vi "Welcome.vi"() -> ()   [LabVIEW 2023]
uses:
  Global/Global 1.vi
  Global/Login Details.vi
  Control/WELCOM SCREEN ENUM.ctl
panel:
  in  "Check 2":bool
  in  "auto":bool
  in  "Test Print":bool
  in  "andon":bool
  in  "MANUAL":bool
  out "error out 2":errorcluster
  in  "error in (no error) 3":errorcluster
  in  "Remove":bool
  in  "Check":bool
  in  "Home":bool
  out "user name":string
  out "STOP":bool
  in  "Tab Control":enum32{"Page 1", "user mangement"}(tab)
  out "Screen Index":i32
  out "error out":errorcluster
  in  "error in (no error)":errorcluster
  in  "LOGIN":bool
  in  "RECIPE":bool
  in  "EXIT":bool
  in  "REPORT":bool
  in  "Hardware Setting":bool
  in  "Shift Setting":bool
  in  "AUTO MODE":bool
  in  "USER MANGMENT":bool
  out "datetime":string
  # "PV Clean Mobility Technologies Traceability System"
  # "USER :"
  # "Powered By - NiVision Automation Systems Pvt. Ltd."
  # "Powered By-Infinity Automation Systems Pvt Ltd. Pune"
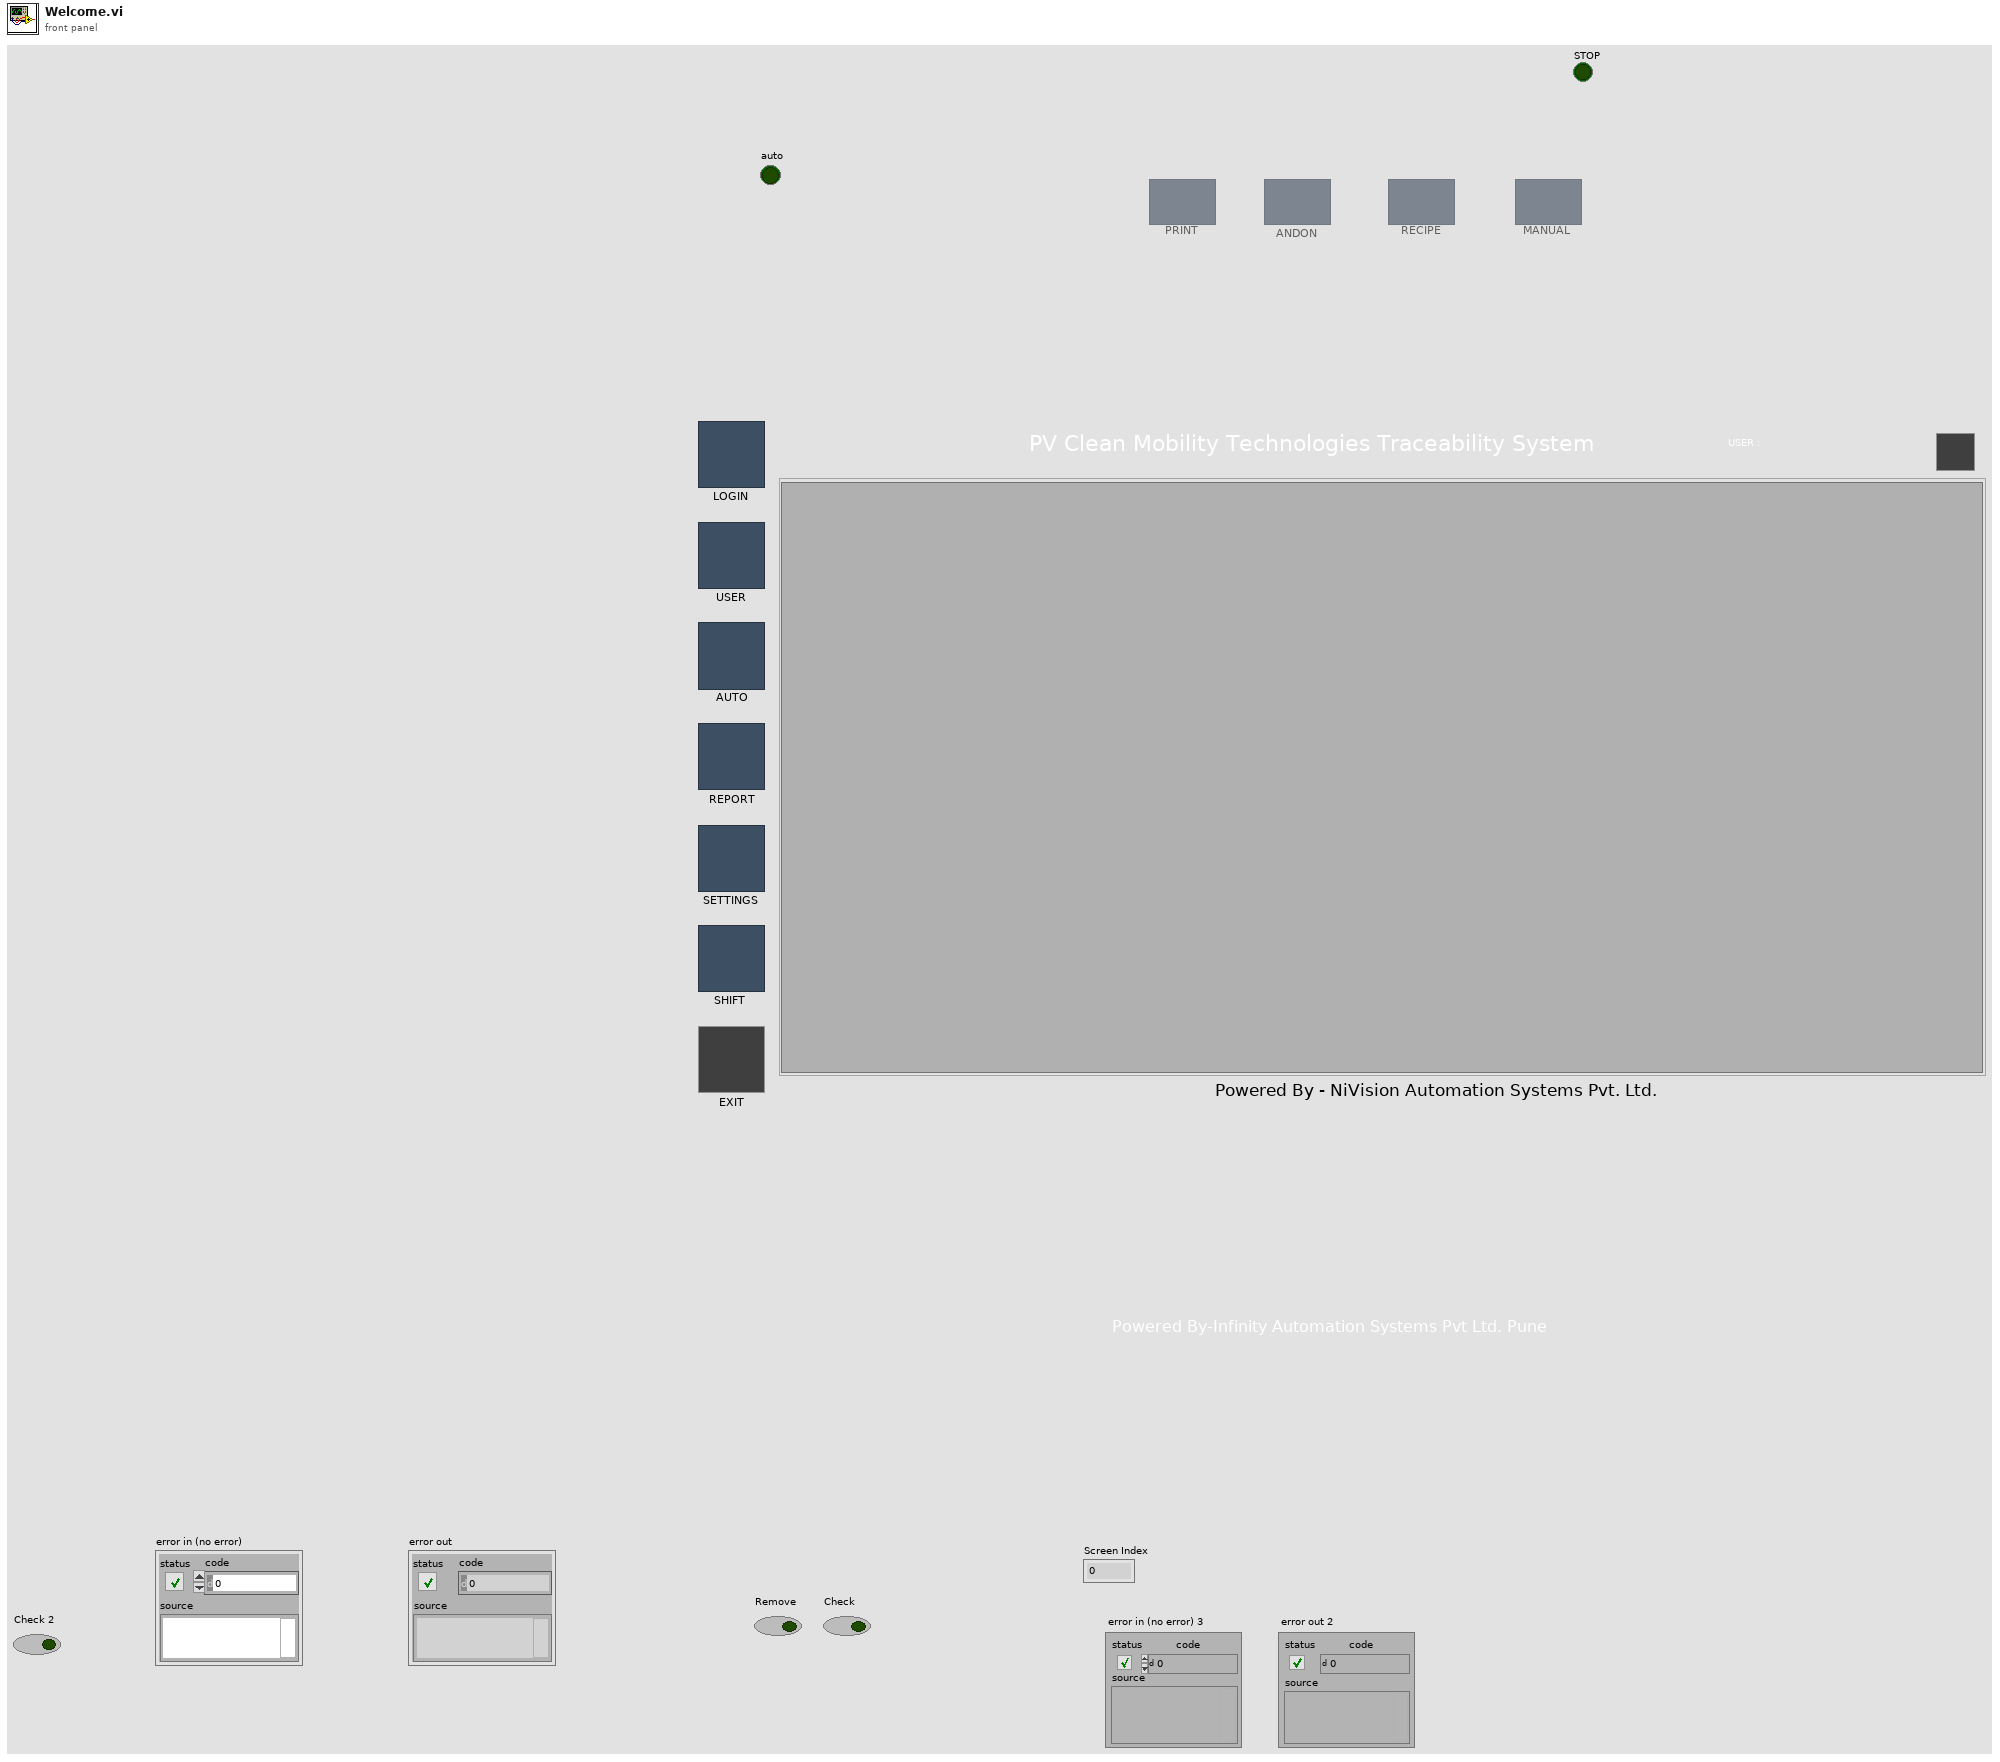
[diagram p1: front panel]
types:
  T1 = typedef "WELCOM SCREEN ENUM.ctl" = enum16{"Initialization", "Wait For Event", "RUN", "LOGIN", "USER MANAGEMENT", "AUTORITY MANAGEMENT", "AUTO MODE", "MANUAL MODE", "BIN MASTER", "CHEMICAL MASTER", "RAW MATERIAL INWARD", "RECIPE INGREDIENT", "REPORT", "SHIFT SETTING", "HARDWARE SETTING", "Check Authority", "TEST PRINT", "EXIT"}
  T2 = cluster{"SCREEN 1":bool, "SCREEN 2":bool, "SCREEN 3":bool, "SCREEN 4":bool, "SCREEN 5":bool, "SCREEN 6":bool, "SCREEN 7":bool, "SCREEN 8":bool, "SCREEN 9":bool, "SCREEN 10":bool, "SCREEN 11":bool, "SCREEN 12":bool, "SCREEN 13":bool, "SCREEN 14":bool, "SCREEN 15":bool, "SCREEN 16":bool, "SCREEN 17":bool, "SCREEN 18":bool, "SCREEN 19":bool, "SCREEN 20":bool}
  T3 = enum8{"Enabled", "Disabled", "Disabled and Grayed Out"}
  T4 = enum32{"Invalid", "Standard", "Closed", "Hidden", "Minimized", "Maximized"}
  T5 = enum32{"Bad", "Idle", "Run top level", "Running"}
  T6 = enum32{"invalid app kind", "Development System", "Run Time System", "Student Edition", "Embedded LabVIEW", "Evaluation", "Custom"}
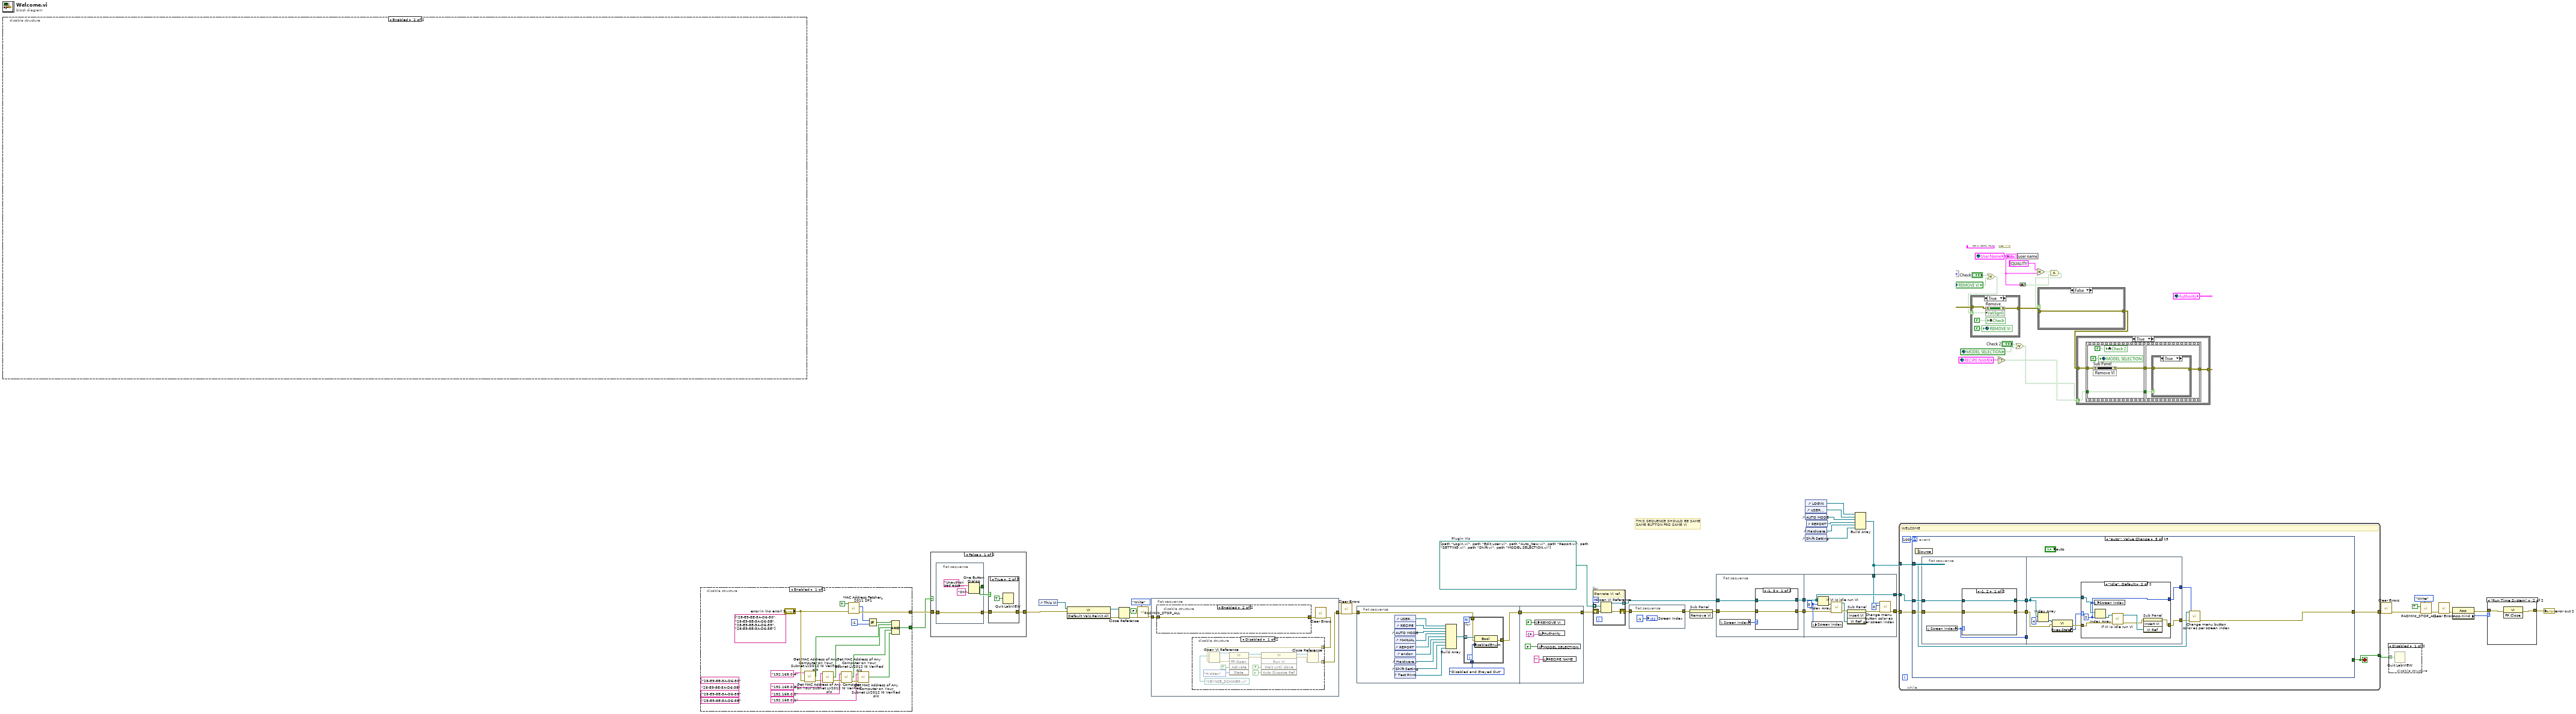
[diagram p0: block diagram]
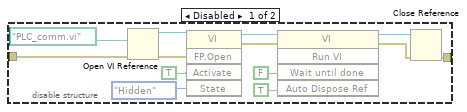
[diagram p2: hidden frame]
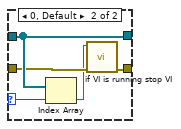
[diagram p4: hidden frame]
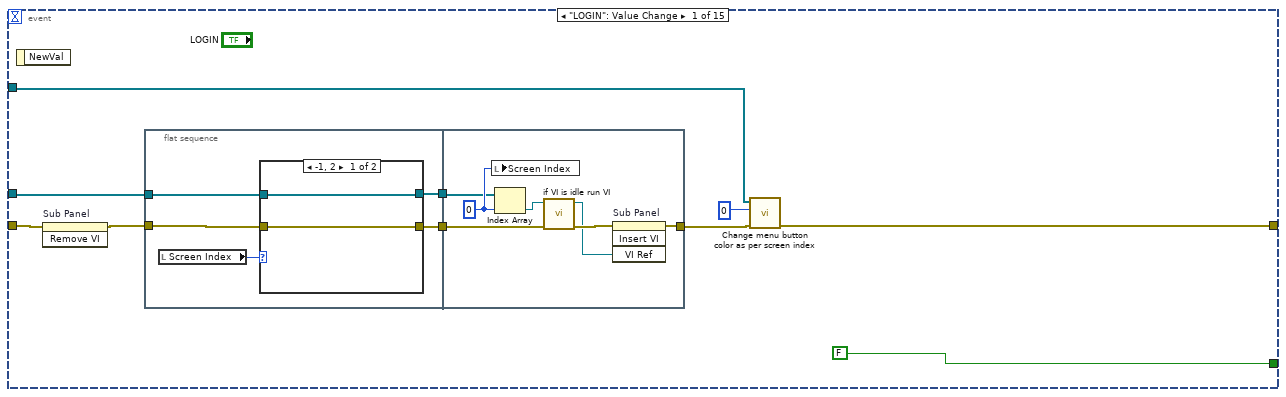
[diagram p7: hidden frame]
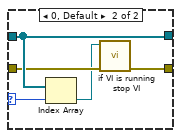
[diagram p8: hidden frame]
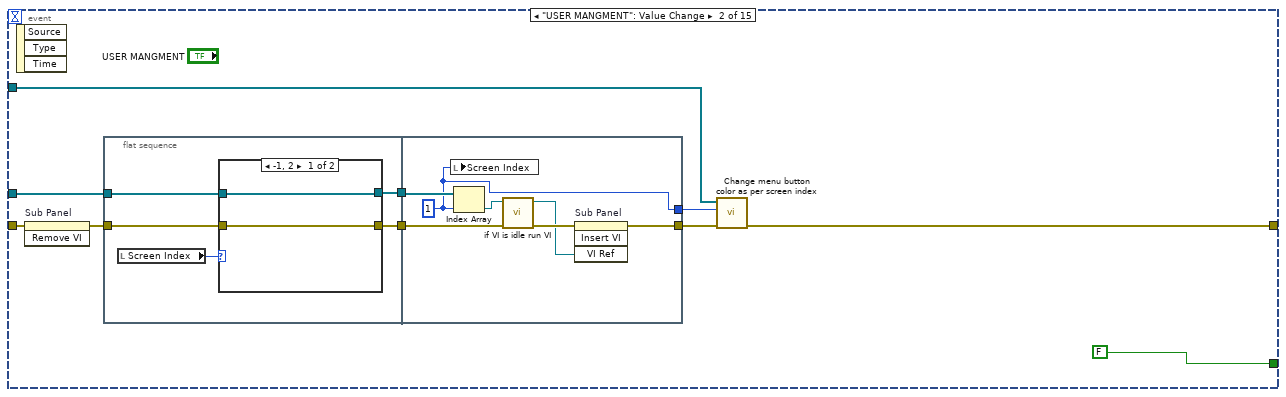
[diagram p9: hidden frame]
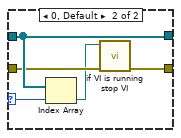
[diagram p10: hidden frame]
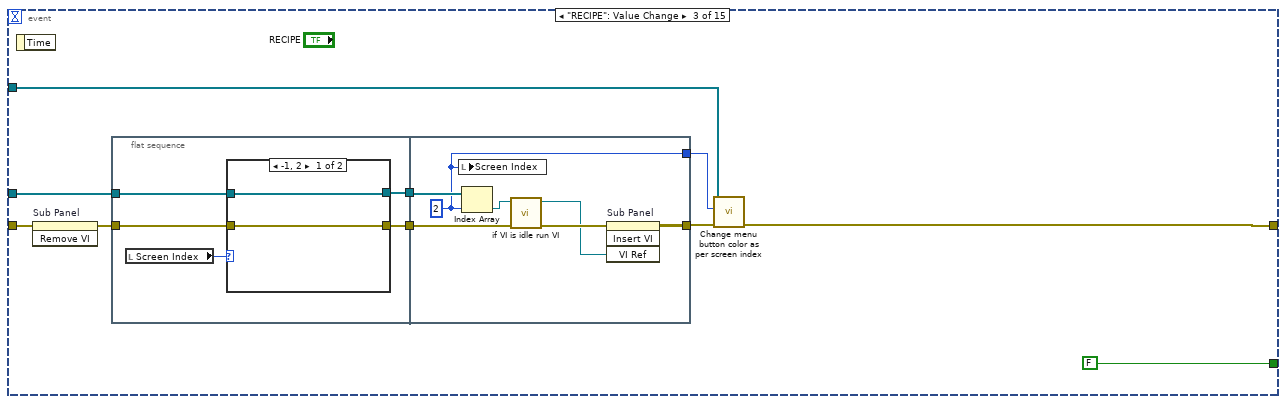
[diagram p11: hidden frame]
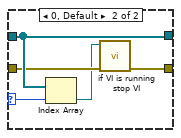
[diagram p12: hidden frame]
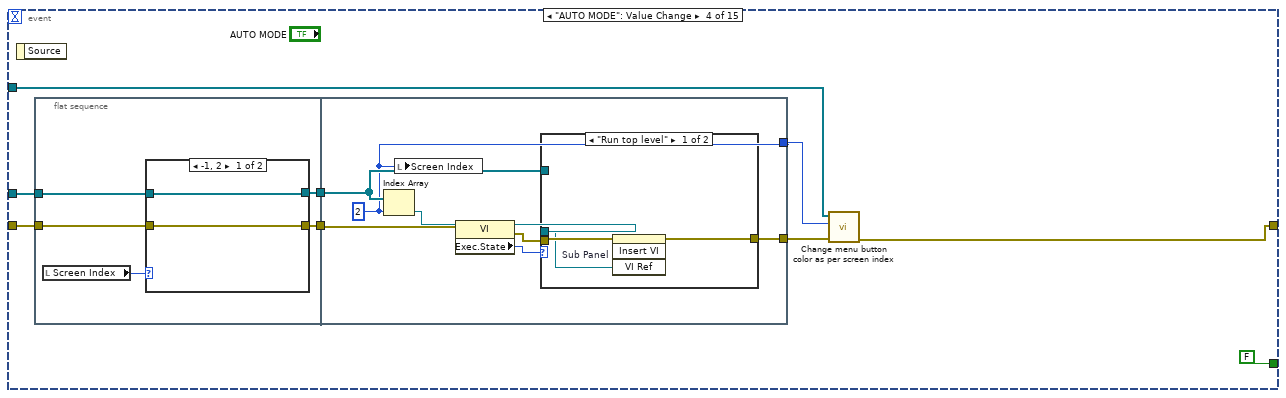
[diagram p13: hidden frame]
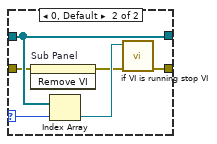
[diagram p14: hidden frame]
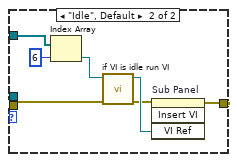
[diagram p15: hidden frame]
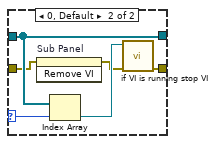
[diagram p16: hidden frame]
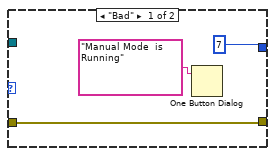
[diagram p17: hidden frame]
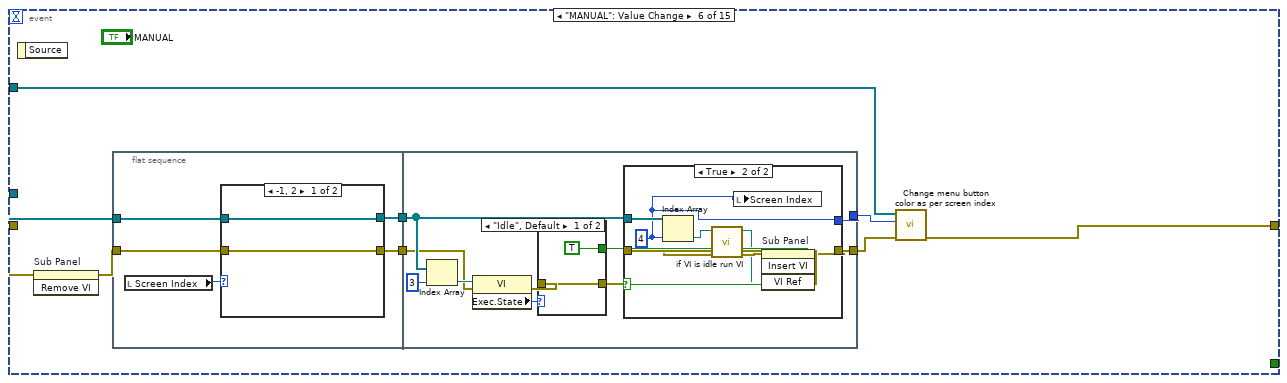
[diagram p18: hidden frame]
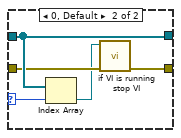
[diagram p19: hidden frame]
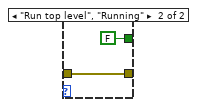
[diagram p20: hidden frame]
diagram:
  w33 = path[] [path "Login.vi", path "Edit user.vi", path "Auto_New.vi", path "Report.vi", path "SETTING.vi", path "Shift.vi", path "MODEL SELECTION.vi"]  # Plugin VIs
  # "THIS SEQUENCE SHOULD BE SAME\nSAME BUTTON FRO SAME VI"
  # "THIS SEQUENCE SHOULD BE SAME\nSAME BUTTON FRO SAME VI"
  n1 = disable-structure shown="Enabled" {
    frame Disabled {
      n2 = flat-sequence {
        tunnel: "error in (no error)" -> [w68]
        tunnel: [w67] -> w43
        frame #0 {
          n3 = invoke class="VI" method="Default Vals.Reinit All"(error in=w68) -> (error out=w67:errorcluster)  [unwired: 2 in, 2 out]
          n4 = global write "Login Details.vi" "Authority"(T2 {"SCREEN 1"=FALSE, "SCREEN 2"=FALSE, "SCREEN 3"=FALSE, "SCREEN 4"=FALSE, "SCREEN 5"=FALSE, "SCREEN 6"=FALSE, "SCREEN 7"=FALSE, "SCREEN 8"=FALSE, "SCREEN 9"=FALSE, "SCREEN 10"=FALSE, "SCREEN 11"=FALSE, "SCREEN 12"=FALSE, "SCREEN 13"=FALSE, "SCREEN 14"=FALSE, "SCREEN 15"=FALSE, "SCREEN 16"=FALSE, "SCREEN 17"=FALSE, "SCREEN 18"=FALSE, "SCREEN 19"=FALSE, "SCREEN 20"=FALSE} ("Authority")) -> ()
        }
      }
      n5 = invoke on="Sub Panel" class="SubPnl" method="Remove VI"(error in=w43) -> (error out=w56:errorcluster)  [unwired: 2 in, 2 out]
      n6 = Open VI Reference(vi path=path "Login.vi", error in (no error)=w56) -> (vi reference=w55:refnum<vi>, error out=w53:errorcluster)  [unwired: 4 in]
      n7 = invoke on="Sub Panel" class="SubPnl" method="Insert VI"(error in=w53, "VI Ref"=w55) -> (error out=w54:errorcluster)  [unwired: 2 in, 3 out]
      n8 = invoke class="VI" method="Run VI"(reference=w55, error in=w54, "Wait until done"=TRUE ("Wait Until Done"), "Auto Dispose Ref"=FALSE ("Auto Dispose Reference")) -> (reference out=w51:refnum<vi>, error out=w52:errorcluster)  [unwired: 1 in, 3 out]
      n9 = Close Reference(reference=w51, error in (no error)=w52) -> (error out=w46:errorcluster)
      n10 = Unbundle By Name(w46) -> ("code"=w50:i32)
      n11 = call <vilib>:"Clear Errors.vi"("error in (no error)"=w46) -> ("error out"=w48:errorcluster)  [unwired: 5 in, 1 out]
      n12 = Not Equal?(x=7, y=w50) -> (x != y?=w49:bool)
      n13 = Select(t=w46, s=w49, f=w48) -> (s? t:f=w47:errorcluster)
      n14 = call <vilib>:"Simple Error Handler.vi"("error in (no error)"=w47) -> ("error out"=w57:errorcluster)  [unwired: 4 in, 4 out]
      n15 = invoke on="Sub Panel" class="SubPnl" method="Remove VI"(error in=w57) -> (error out=w45:errorcluster)  [unwired: 2 in, 2 out]
      n16 = while {
        tunnel: w45 -> [w75]
        shift-right: [w77] -> _
        shift-left: WELCOM_SCREEN_ENUM."Initialization" -> [w71]
        shift-right: [w74] -> _
        shift-left: cluster{"VI Run":string} {"VI Run"=""} -> [w73]
        tunnel: [w76] -> w63
        stop <- w72 stop-if-true
        n17 = case shown="\"AUTORITY MANAGEMENT\"" w71 {
          tunnel: [WELCOM_SCREEN_ENUM."Check Authority" w102 WELCOM_SCREEN_ENUM."Wait For Event" WELCOM_SCREEN_ENUM."Wait For Event" WELCOM_SCREEN_ENUM."RUN" WELCOM_SCREEN_ENUM."RUN" WELCOM_SCREEN_ENUM."RUN" WELCOM_SCREEN_ENUM."RUN" WELCOM_SCREEN_ENUM."RUN" WELCOM_SCREEN_ENUM."RUN" WELCOM_SCREEN_ENUM."RUN" WELCOM_SCREEN_ENUM."RUN" WELCOM_SCREEN_ENUM."RUN" WELCOM_SCREEN_ENUM."RUN" WELCOM_SCREEN_ENUM."RUN" WELCOM_SCREEN_ENUM."RUN" WELCOM_SCREEN_ENUM."RUN" w229] -> w77
          tunnel: [w95 w101 w123 w127 w133 w139 w145 w151 w157 w163 w169 w175 w181 w187 w193 w199 w205 w224] -> w76
          tunnel: w75 -> [w95 w101 w123 w127 w133 w139 w145 w151 w157 w163 w169 w175 w181 w187 w193 w199 w205 w223]
          tunnel: [w93 w99 w122 w126 w131 w137 w142 w146 w155 w161 w167 w170 w177 w185 w188 w194 w203 w222] -> w74
          tunnel: w73 -> [w93 w99 w122 w126 w132 w138 w143 w147 w156 w162 w168 w171 w178 w186 w189 w195 w204 w222]
          tunnel: [FALSE FALSE FALSE TRUE FALSE FALSE FALSE FALSE FALSE FALSE FALSE FALSE FALSE FALSE FALSE FALSE FALSE FALSE] -> w72
          frame "Initialization", Default {
            n18 = control-ref of="USER MANGMENT"() -> (w80:refnum<vi>)
            n19 = control-ref of="RECIPE"() -> (w81:refnum<vi>)
            n20 = control-ref of="AUTO MODE"() -> (w82:refnum<vi>)
            n21 = control-ref of="REPORT"() -> (w88:refnum<vi>)
            n22 = control-ref of="Shift Setting"() -> (w89:refnum<vi>)
            n23 = control-ref of="Hardware Setting"() -> (w90:refnum<vi>)
            n24 = Build Array(w80, w81, w82, w88, w89, w90) -> (w79:refnum<vi>[], w83:refnum<vi>, w84:refnum<vi>, w85:refnum<vi>, w86:refnum<vi>, w87:refnum<vi>, w91:refnum<vi>)
            n25 = for {
              tunnel: w79 -> [w97] mode=indexing
              n26 = property class="Bool"(reference=w97, "DisabledEnum"=T3."Disabled and Grayed Out" ("Disabled")) -> ()  [unwired: 1 in, 2 out]
            }
          }
          frame "Wait For Event" {
            n27 = Search 1D Array(1D array=bool[] [], element=TRUE) -> (index of element=w104:i32)  [unwired: 1 in]
            n28 = case shown="11" w104 {
              tunnel: [WELCOM_SCREEN_ENUM."Wait For Event" WELCOM_SCREEN_ENUM."EXIT" WELCOM_SCREEN_ENUM."LOGIN" WELCOM_SCREEN_ENUM."USER MANAGEMENT" WELCOM_SCREEN_ENUM."AUTORITY MANAGEMENT" WELCOM_SCREEN_ENUM."AUTO MODE" WELCOM_SCREEN_ENUM."MANUAL MODE" WELCOM_SCREEN_ENUM."BIN MASTER" WELCOM_SCREEN_ENUM."CHEMICAL MASTER" WELCOM_SCREEN_ENUM."RAW MATERIAL INWARD" WELCOM_SCREEN_ENUM."REPORT" WELCOM_SCREEN_ENUM."SHIFT SETTING" WELCOM_SCREEN_ENUM."HARDWARE SETTING" WELCOM_SCREEN_ENUM."TEST PRINT" WELCOM_SCREEN_ENUM."RECIPE INGREDIENT"] -> w102
              frame -1, Default {
              }
              frame 0 {
              }
              frame 1 {
              }
              frame 2 {
              }
              frame 3 {
              }
              frame 4 {
              }
              frame 5 {
              }
              frame 6 {
              }
              frame 7 {
              }
              frame 8 {
              }
              frame 9 {
              }
              frame 10 {
              }
              frame 11 {
              }
              frame 12 {
              }
              frame 13 {
              }
            }
          }
          frame "Check Authority" {
          }
          frame "EXIT" {
          }
          frame "LOGIN" {
            w130 = "Login.vi"  # VI Run
            n29 = Bundle By Name(cluster=w132, "VI Run"=w130) -> (w131:cluster{"VI Run":string})
          }
          frame "USER MANAGEMENT" {
            w136 = "User Management.vi"  # VI Run
            n30 = Bundle By Name(cluster=w138, "VI Run"=w136) -> (w137:cluster{"VI Run":string})
          }
          frame "AUTORITY MANAGEMENT" {
            w141 = "Authority Management.vi"  # VI Run
            n31 = Bundle By Name(cluster=w143, "VI Run"=w141) -> (w142:cluster{"VI Run":string})
          }
          frame "AUTO MODE" {
            w148 = "AUTO MODE.vi"  # VI Run
            n32 = Bundle By Name(cluster=w147, "VI Run"=w148) -> (w146:cluster{"VI Run":string})
          }
          frame "MANUAL MODE" {
            w154 = "Manual Mode.vi"  # VI Run
            n33 = Bundle By Name(cluster=w156, "VI Run"=w154) -> (w155:cluster{"VI Run":string})
          }
          frame "BIN MASTER" {
            w160 = "Bin Master.vi"  # VI Run
            n34 = Bundle By Name(cluster=w162, "VI Run"=w160) -> (w161:cluster{"VI Run":string})
          }
          frame "CHEMICAL MASTER" {
            w166 = "Chemical Master.vi"  # VI Run
            n35 = Bundle By Name(cluster=w168, "VI Run"=w166) -> (w167:cluster{"VI Run":string})
          }
          frame "RAW MATERIAL INWARD" {
            w172 = "raw material inward.vi"  # VI Run
            n36 = Bundle By Name(cluster=w171, "VI Run"=w172) -> (w170:cluster{"VI Run":string})
          }
          frame "RECIPE INGREDIENT" {
            w179 = "Recipe_Ingredients.vi"  # VI Run
            n37 = Bundle By Name(cluster=w178, "VI Run"=w179) -> (w177:cluster{"VI Run":string})
          }
          frame "REPORT" {
            w184 = "Report.vi"  # VI Run
            n38 = Bundle By Name(cluster=w186, "VI Run"=w184) -> (w185:cluster{"VI Run":string})
          }
          frame "SHIFT SETTING" {
            w190 = "shift setting.vi"  # VI Run
            n39 = Bundle By Name(cluster=w189, "VI Run"=w190) -> (w188:cluster{"VI Run":string})
          }
          frame "HARDWARE SETTING" {
            w196 = "Hardware Setting.vi"  # VI Run
            n40 = Bundle By Name(cluster=w195, "VI Run"=w196) -> (w194:cluster{"VI Run":string})
          }
          frame "TEST PRINT" {
            w202 = "Test Print.vi"  # VI Run
            n41 = Bundle By Name(cluster=w204, "VI Run"=w202) -> (w203:cluster{"VI Run":string})
          }
          frame "RUN" {
            w230 = "Login.vi"  # x
            n42 = Unbundle By Name(w222) -> ("VI Run"=w231:string)
            n43 = invoke on="Sub Panel" class="SubPnl" method="Remove VI"(error in=w223) -> (error out=w212:errorcluster)  [unwired: 2 in, 2 out]
            n44 = Equal?(x=w230, y=w231) -> (x = y?=w228:bool)
            n45 = String To Path(string=w231) -> (path=w207:path)
            n46 = Open VI Reference(vi path=w207, error in (no error)=w212) -> (vi reference=w213:refnum<vi>, error out=w215:errorcluster)  [unwired: 4 in]
            n47 = invoke on="Sub Panel" class="SubPnl" method="Insert VI"(error in=w215, "VI Ref"=w213) -> (error out=w214:errorcluster)  [unwired: 2 in, 3 out]
            n48 = invoke class="VI" method="Run VI"(reference=w213, error in=w214, "Wait until done"=TRUE ("Wait Until Done"), "Auto Dispose Ref"=FALSE ("Auto Dispose Reference")) -> (reference out=w217:refnum<vi>, error out=w216:errorcluster)  [unwired: 1 in, 3 out]
            n49 = Close Reference(reference=w217, error in (no error)=w216) -> (error out=w206:errorcluster)
            n50 = Unbundle By Name(w206) -> ("code"=w218:i32)
            n51 = call <vilib>:"Clear Errors.vi"("error in (no error)"=w206) -> ("error out"=w220:errorcluster)  [unwired: 5 in, 1 out]
            n52 = Not Equal?(x=7, y=w218) -> (x != y?=w219:bool)
            n53 = Select(t=WELCOM_SCREEN_ENUM."Check Authority", s=w228, f=WELCOM_SCREEN_ENUM."Wait For Event") -> (s? t:f=w229:T1)
            n54 = Select(t=w206, s=w219, f=w220) -> (s? t:f=w221:errorcluster)
            n55 = call <vilib>:"Simple Error Handler.vi"("error in (no error)"=w221) -> ("error out"=w211:errorcluster)  [unwired: 4 in, 4 out]
            n56 = invoke on="Sub Panel" class="SubPnl" method="Remove VI"(error in=w211) -> (error out=w224:errorcluster)  [unwired: 2 in, 2 out]
          }
        }
        "STOP" <- w72
        n57 = Wait (ms)(milliseconds to wait=u32 100) -> ()  [unwired: 1 out]
      }
      n58 = while {
        tunnel: w43 -> [w65]
        tunnel: [w65] -> w41
        stop <- w66 stop-if-true
        n59 = local read "STOP"() -> (w66:bool)
      }
      n60 = Merge Errors(w41, w63) -> (→"error out":errorcluster)
      n61 = disable-structure shown="Enabled" {
        disable-tunnel: w63 -> [w70 _]
        frame Enabled {
          n62 = invoke class="VI" method="FP.Close"(error in=w70) -> ()  [unwired: 2 in, 3 out]
        }
        frame Disabled {
        }
      }
    }
    frame Enabled {
    }
  }
  n63 = disable-structure shown="Enabled" {
    disable-tunnel: [w248 _] -> w4
    disable-tunnel: [w236 TRUE] -> w2
    frame Enabled {
      (unwired) string[] ["28-E9-8E-5A-D6-50", "28-E9-8E-5A-D6-3B", "28-E9-8E-5A-D6-59", "28-E9-8E-5A-D6-5E"]
      (unwired) "28-E9-8E-5A-D6-5E" ("IP Address")
      (unwired) "28-E9-8E-5A-D6-59" ("IP Address")
      (unwired) "28-E9-8E-5A-D6-3B" ("IP Address")
      (unwired) "28-E9-8E-5A-D6-50" ("IP Address")
      n64 = call "Get MAC Address of Any Computer on Your Subnet LV2012 NI Verified plc.vi"("error constant"="error in (no error) 3", "IP Address"="192.168.0.4") -> ("error out"=w244:errorcluster, "x .and. y?"=w235:bool)  [unwired: 1 in, 1 out]
      n65 = call "Get MAC Address of Any Computer on Your Subnet LV2012 NI Verified plc.vi"("error constant"=w244, "IP Address"="192.168.0.3") -> ("error out"=w242:errorcluster, "x .and. y?"=w234:bool)  [unwired: 1 in, 1 out]
      n66 = call "Get MAC Address of Any Computer on Your Subnet LV2012 NI Verified plc.vi"("error constant"=w242, "IP Address"="192.168.0.2") -> ("error out"=w243:errorcluster, "x .and. y?"=w233:bool)  [unwired: 1 in, 1 out]
      n67 = call "MAC Address Fetcher_2011 SP1.vi"("error in (no error)"="error in (no error) 3", "Search all adapters?"=TRUE) -> ("error out"=w248:errorcluster, "index of element"=w239:i32)  [unwired: 6 in, 2 out]
      n68 = call "Get MAC Address of Any Computer on Your Subnet LV2012 NI Verified plc.vi"("error constant"=w243, "IP Address"="192.168.0.1") -> ("x .and. y?"=w232:bool)  [unwired: 1 in, 2 out]
      n69 = Not Equal?(x=w239, y=-1) -> (x != y?=w237:bool)
      n70 = Compound Arithmetic op=AND(w237, w235, w234, w233, w232) -> (w236:bool)
    }
    frame Disabled {
    }
  }
  n71 = case shown="False" w2 {
    tunnel: w4 -> [w252 w262]
    tunnel: [w251 w262] -> w3
    frame False {
      n72 = flat-sequence {
        tunnel: [w257] -> w254
        tunnel: [w256] -> w253
        tunnel: w252 -> [w256]
        frame #0 {
          n73 = One Button Dialog(message="Unauthorised access to this system\nPlease contact to NIVision Automation Systems Pvt Ltd", button name ("OK")="OK") -> (true=w257:bool)
        }
      }
      n74 = case shown="True" w254 {
        tunnel: w253 -> [w259 w260]
        tunnel: [w259 w260] -> w251
        frame False {
        }
        frame True {
          n75 = Quit LabVIEW(quit? (T)=TRUE) -> ()
        }
      }
    }
    frame True {
    }
  }
  n76 = control-ref of="This VI"() -> (w40:refnum<vi>)
  n77 = invoke class="VI" method="Default Vals.Reinit All"(reference=w40, error in=w3) -> (reference out=w38:refnum<vi>, error out=w39:errorcluster)  [unwired: 1 in, 1 out]
  n78 = Close Reference(reference=w38, error in (no error)=w39) -> (error out=w6:errorcluster)
  n79 = call "PADMINI_STOP_ALL.vi"("Enum"=enum16{"Read", "Write"}."Write", "error in (no error)"=w6, "Boolean"=FALSE) -> ("error out"=w5:errorcluster)  [unwired: 7 in, 1 out]
  n80 = flat-sequence {
    tunnel: w5 -> [w266]
    tunnel: [w263] -> w21
    frame #0 {
      n81 = disable-structure shown="Enabled" {
        disable-tunnel: w266 -> [w271 w280]
        disable-tunnel: [w267 w280] -> w265
        frame Disabled {
          n82 = Open VI Reference(vi path=path "PLC_comm.vi", error in (no error)=w271) -> (vi reference=w273:refnum<vi>, error out=w274:errorcluster)  [unwired: 4 in]
          n83 = invoke class="VI" method="FP.Open"(reference=w273, error in=w274, "Activate"=TRUE ("Activate?"), "State"=T4."Hidden") -> (reference out=w276:refnum<vi>, error out=w275:errorcluster)  [unwired: 1 in, 3 out]
          n84 = invoke class="VI" method="Run VI"(reference=w276, error in=w275, "Wait until done"=FALSE ("Wait Until Done"), "Auto Dispose Ref"=TRUE ("Auto Dispose Reference")) -> (reference out=w270:refnum<vi>, error out=w269:errorcluster)  [unwired: 1 in, 3 out]
          n85 = Close Reference(reference=w270, error in (no error)=w269) -> (error out=w267:errorcluster)
        }
        frame Enabled {
        }
      }
      n86 = call <vilib>:"Clear Errors.vi"("error in (no error)"=w265) -> ("error out"=w264:errorcluster)  [unwired: 5 in, 1 out]
      n87 = disable-structure shown="Disabled" {
        disable-tunnel: w264 -> [w283 w294]
        disable-tunnel: [w282 w294] -> w263
        frame Disabled {
          n88 = Open VI Reference(vi path=path "KEYNCE_SCANNER.vi", error in (no error)=w283) -> (vi reference=w290:refnum<vi>, error out=w289:errorcluster)  [unwired: 4 in]
          n89 = invoke class="VI" method="FP.Open"(reference=w290, error in=w289, "Activate"=TRUE ("Activate?"), "State"=T4."Hidden") -> (reference out=w287:refnum<vi>, error out=w288:errorcluster)  [unwired: 1 in, 3 out]
          n90 = invoke class="VI" method="Run VI"(reference=w287, error in=w288, "Wait until done"=FALSE ("Wait Until Done"), "Auto Dispose Ref"=TRUE ("Auto Dispose Reference")) -> (reference out=w291:refnum<vi>, error out=w292:errorcluster)  [unwired: 1 in, 3 out]
          n91 = Close Reference(reference=w291, error in (no error)=w292) -> (error out=w282:errorcluster)
        }
        frame Enabled {
        }
      }
    }
  }
  n92 = call <vilib>:"Clear Errors.vi"("error in (no error)"=w21) -> ("error out"=w20:errorcluster)  [unwired: 5 in, 1 out]
  n93 = flat-sequence {
    tunnel: w20 -> [w296]
    tunnel: [w295] -> w13
    tunnel: [w316] -> w23
    tunnel: w13 -> [w316]
    frame #0 {
      n94 = control-ref of="Shift Setting"() -> (w300:refnum<vi>)
      n95 = control-ref of="Test Print"() -> (w299:refnum<vi>)
      n96 = control-ref of="USER MANGMENT"() -> (w307:refnum<vi>)
      n97 = control-ref of="RECIPE"() -> (w306:refnum<vi>)
      n98 = control-ref of="AUTO MODE"() -> (w305:refnum<vi>)
      n99 = control-ref of="MANUAL"() -> (w304:refnum<vi>)
      n100 = control-ref of="REPORT"() -> (w303:refnum<vi>)
      n101 = control-ref of="andon"() -> (w302:refnum<vi>)
      n102 = control-ref of="Hardware Setting"() -> (w301:refnum<vi>)
      n103 = Build Array(w307, w306, w305, w304, w303, w302, w301, w300, w299) -> (w298:refnum<vi>[])
      n104 = for {
        tunnel: w298 -> [w311] mode=indexing
        tunnel: w296 -> [w310]
        tunnel: T3."Disabled and Grayed Out" ("Disabled") -> [w309]
        tunnel: [w308] -> w295
        n105 = property class="Bool"(reference=w311, error in=w310, "DisabledEnum"=w309) -> (error out=w308:errorcluster)  [unwired: 1 out]
      }
    }
    frame #1 {
      n106 = global write "Global 1.vi" "REMOVE VI"(FALSE ("REMOVE VI")) -> ()
      n107 = global write "Global 1.vi" "MODEL SELECTION"(FALSE ("REMOVE VI")) -> ()
      n108 = global write "Login Details.vi" "Authority"(T2 {"SCREEN 1"=FALSE, "SCREEN 2"=FALSE, "SCREEN 3"=FALSE, "SCREEN 4"=FALSE, "SCREEN 5"=FALSE, "SCREEN 6"=FALSE, "SCREEN 7"=FALSE, "SCREEN 8"=FALSE, "SCREEN 9"=FALSE, "SCREEN 10"=FALSE, "SCREEN 11"=FALSE, "SCREEN 12"=FALSE, "SCREEN 13"=FALSE, "SCREEN 14"=FALSE, "SCREEN 15"=FALSE, "SCREEN 16"=FALSE, "SCREEN 17"=FALSE, "SCREEN 18"=FALSE, "SCREEN 19"=FALSE, "SCREEN 20"=FALSE} ("Authority")) -> ()
      n109 = global write "Global 1.vi" "RECIPE NAME"("" ("RECIPE NAME")) -> ()
    }
  }
  n110 = for {
    tunnel: w33 -> [w318] mode=indexing
    tunnel: [w319] -> w26 mode=indexing
    shift-right: [w320] -> w32
    shift-left: w23 -> [w317]
    # "Genrate VI ref."
    n111 = Open VI Reference(vi path=w318, error in (no error)=w317) -> (vi reference=w319:refnum<vi>, error out=w320:errorcluster)  [unwired: 4 in]
  }
  n112 = flat-sequence {
    tunnel: w32 -> [w322]
    tunnel: [w322] -> w28
    frame #0 {
      "Screen Index" <- -1 ("Screen Index")
    }
  }
  n113 = invoke on="Sub Panel" class="SubPnl" method="Remove VI"(error in=w28) -> (error out=w29:errorcluster)  [unwired: 2 in, 2 out]
  n114 = flat-sequence {
    tunnel: w26 -> [w325]
    tunnel: [w327] -> w31
    tunnel: [w324] -> w30
    tunnel: w29 -> [w323]
    tunnel: w31 -> [w343]
    tunnel: w30 -> [w339]
    tunnel: [w336] -> w27
    tunnel: [w339] -> w25
    tunnel: w24 -> [w335]
    frame #0 {
      n115 = local read "Screen Index"() -> (w326:i32)
      n116 = case shown="-1, 3" w326 {
        selector: w326 -> [_ w334]
        tunnel: w323 -> [w329 w332]
        tunnel: [w329 w331] -> w327
        tunnel: w325 -> [w328 w333]
        tunnel: [w328 w333] -> w324
        frame -1, 3 {
        }
        frame 0, Default {
          n117 = Index Array(array=w333, index=w334) -> (element=w330:refnum<vi>)
          n118 = call "if VI is running stop VI.vi"("error in (no error)"=w332, "VI in"=w330) -> ("error out"=w331:errorcluster)  [unwired: 8 in, 1 out]
        }
      }
    }
    frame #1 {
      w344 = 0 ("index")
      n119 = local write "Screen Index"(w344) -> ()
      n120 = Index Array(array=w339, index=w344) -> (element=w342:refnum<vi>)
      n121 = call "if VI is idle run VI.vi"("error in (no error)"=w343, "VI in"=w342) -> ("error out"=w341:errorcluster, "VI out"=w340:refnum<vi>)  [unwired: 8 in]
      n122 = invoke on="Sub Panel" class="SubPnl" method="Insert VI"(error in=w341, "VI Ref"=w340) -> (error out=w337:errorcluster)  [unwired: 2 in, 3 out]
      n123 = call "Change menu button color as per screen index.vi"("error in (no error)"=w337, "Screen Index"=0, "Array"=w335) -> ("error out"=w336:errorcluster)  [unwired: 8 in]
    }
  }
  n124 = control-ref of="LOGIN"() -> (w19:refnum<vi>)
  n125 = control-ref of="USER MANGMENT"() -> (w18:refnum<vi>)
  n126 = control-ref of="AUTO MODE"() -> (w17:refnum<vi>)
  n127 = control-ref of="Shift Setting"() -> (w14:refnum<vi>)
  n128 = control-ref of="Hardware Setting"() -> (w15:refnum<vi>)
  n129 = control-ref of="REPORT"() -> (w16:refnum<vi>)
  n130 = Build Array(w19, w18, w17, w16, w15, w14) -> (w24:refnum<vi>[])
  n131 = while {
    tunnel: w27 -> [w347]
    tunnel: [w349] -> w22
    tunnel: w25 -> [w346]
    tunnel: w24 -> [w348]
    tunnel: [w345] -> w1
    stop <- w345 stop-if-true
    # "WELCOME"
    n132 = event shown="[4] \"auto\": Value Change" {
      selector: _ -> [_ _ _ _ _ _ _ _ _ _ _ _ _ _ _]
      dyn-events: _ -> [_ _ _ _ _ _ _ _ _ _ _ _ _ _ _]
      timeout: 100 -> [_ _ _ _ _ _ _ _ _ _ _ _ _ _ _]
      tunnel: [FALSE FALSE FALSE FALSE _ _ FALSE FALSE FALSE FALSE FALSE FALSE w715 FALSE FALSE] -> w345
      tunnel: [w353 w384 w413 w445 w478 w518 w567 w596 w625 w654 w683 w710 w714 w755 w758] -> w349
      tunnel: w346 -> [w359 w388 w417 w441 w482 w521 w571 w600 w629 w658 w687 _ w716 _ _]
      tunnel: w348 -> [w352 w382 w410 w444 w481 w519 w565 w593 w622 w652 w680 w709 w719 w753 _]
      tunnel: w347 -> [w351 w380 w409 w440 w483 w520 w563 w592 w621 w650 w679 w708 w723 w752 w770]
      event "LOGIN": Value Change {
        n133 = event-data() -> ()  [unwired: 1 in, 1 out]
        n134 = invoke on="Sub Panel" class="SubPnl" method="Remove VI"(error in=w351) -> (error out=w356:errorcluster)  [unwired: 2 in, 2 out]
        n135 = flat-sequence {
          tunnel: w359 -> [w363]
          tunnel: [w365] -> w358
          tunnel: [w362] -> w357
          tunnel: w356 -> [w361]
          tunnel: w358 -> [w377]
          tunnel: w357 -> [w378]
          tunnel: [w373] -> w354
          frame #0 {
            n136 = local read "Screen Index"() -> (w364:i32)
            n137 = case shown="-1, 2" w364 {
              selector: w364 -> [_ w372]
              tunnel: w361 -> [w367 w370]
              tunnel: [w367 w369] -> w365
              tunnel: w363 -> [w366 w371]
              tunnel: [w366 w371] -> w362
              frame -1, 2 {
              }
              frame 0, Default {
                n138 = Index Array(array=w371, index=w372) -> (element=w368:refnum<vi>)
                n139 = call "if VI is running stop VI.vi"("error in (no error)"=w370, "VI in"=w368) -> ("error out"=w369:errorcluster)  [unwired: 8 in, 1 out]
              }
            }
          }
          frame #1 {
            w379 = 0 ("index")
            n140 = local write "Screen Index"(w379) -> ()
            n141 = Index Array(array=w378, index=w379) -> (element=w376:refnum<vi>)
            n142 = call "if VI is idle run VI.vi"("error in (no error)"=w377, "VI in"=w376) -> ("error out"=w375:errorcluster, "VI out"=w374:refnum<vi>)  [unwired: 8 in]
            n143 = invoke on="Sub Panel" class="SubPnl" method="Insert VI"(error in=w375, "VI Ref"=w374) -> (error out=w373:errorcluster)  [unwired: 2 in, 3 out]
          }
        }
        n144 = call "Change menu button color as per screen index.vi"("error in (no error)"=w354, "Screen Index"=0, "Array"=w352) -> ("error out"=w353:errorcluster)  [unwired: 8 in]
      }
      event "USER MANGMENT": Value Change {
        n145 = event-data() -> ()  [unwired: 1 in, 3 out]
        n146 = invoke on="Sub Panel" class="SubPnl" method="Remove VI"(error in=w380) -> (error out=w385:errorcluster)  [unwired: 2 in, 2 out]
        n147 = flat-sequence {
          tunnel: w385 -> [w394]
          tunnel: w388 -> [w391]
          tunnel: [w393] -> w387
          tunnel: [w390] -> w386
          tunnel: [w407] -> w383
          tunnel: w387 -> [w406]
          tunnel: w386 -> [w408]
          tunnel: [w402] -> w381
          frame #0 {
            n148 = local read "Screen Index"() -> (w392:i32)
            n149 = case shown="-1, 2" w392 {
              selector: w392 -> [_ w401]
              tunnel: w394 -> [w396 w399]
              tunnel: [w396 w398] -> w393
              tunnel: w391 -> [w395 w400]
              tunnel: [w395 w400] -> w390
              frame -1, 2 {
              }
              frame 0, Default {
                n150 = Index Array(array=w400, index=w401) -> (element=w397:refnum<vi>)
                n151 = call "if VI is running stop VI.vi"("error in (no error)"=w399, "VI in"=w397) -> ("error out"=w398:errorcluster)  [unwired: 8 in, 1 out]
              }
            }
          }
          frame #1 {
            w402 = 1 ("index")
            n152 = local write "Screen Index"(w402) -> ()
            n153 = Index Array(array=w408, index=w402) -> (element=w404:refnum<vi>)
            n154 = call "if VI is idle run VI.vi"("error in (no error)"=w406, "VI in"=w404) -> ("error out"=w405:errorcluster, "VI out"=w403:refnum<vi>)  [unwired: 8 in]
            n155 = invoke on="Sub Panel" class="SubPnl" method="Insert VI"(error in=w405, "VI Ref"=w403) -> (error out=w407:errorcluster)  [unwired: 2 in, 3 out]
          }
        }
        n156 = call "Change menu button color as per screen index.vi"("error in (no error)"=w383, "Screen Index"=w381, "Array"=w382) -> ("error out"=w384:errorcluster)  [unwired: 8 in]
      }
      event "RECIPE": Value Change {
        n157 = event-data() -> ()  [unwired: 1 in, 1 out]
        n158 = invoke on="Sub Panel" class="SubPnl" method="Remove VI"(error in=w409) -> (error out=w414:errorcluster)  [unwired: 2 in, 2 out]
        n159 = flat-sequence {
          tunnel: w414 -> [w423]
          tunnel: w417 -> [w420]
          tunnel: [w422] -> w416
          tunnel: [w419] -> w415
          tunnel: [w436] -> w412
          tunnel: w416 -> [w435]
          tunnel: w415 -> [w437]
          tunnel: [w431] -> w411
          frame #0 {
            n160 = local read "Screen Index"() -> (w421:i32)
            n161 = case shown="-1, 2" w421 {
              selector: w421 -> [_ w430]
              tunnel: w423 -> [w425 w428]
              tunnel: [w425 w427] -> w422
              tunnel: w420 -> [w424 w429]
              tunnel: [w424 w429] -> w419
              frame -1, 2 {
              }
              frame 0, Default {
                n162 = Index Array(array=w429, index=w430) -> (element=w426:refnum<vi>)
                n163 = call "if VI is running stop VI.vi"("error in (no error)"=w428, "VI in"=w426) -> ("error out"=w427:errorcluster)  [unwired: 8 in, 1 out]
              }
            }
          }
          frame #1 {
            w431 = 2 ("index")
            n164 = local write "Screen Index"(w431) -> ()
            n165 = Index Array(array=w437, index=w431) -> (element=w432:refnum<vi>)
            n166 = call "if VI is idle run VI.vi"("error in (no error)"=w435, "VI in"=w432) -> ("error out"=w434:errorcluster, "VI out"=w433:refnum<vi>)  [unwired: 8 in]
            n167 = invoke on="Sub Panel" class="SubPnl" method="Insert VI"(error in=w434, "VI Ref"=w433) -> (error out=w436:errorcluster)  [unwired: 2 in, 3 out]
          }
        }
        n168 = call "Change menu button color as per screen index.vi"("error in (no error)"=w412, "Screen Index"=w411, "Array"=w410) -> ("error out"=w413:errorcluster)  [unwired: 8 in]
      }
      event "AUTO MODE": Value Change {
        n169 = event-data() -> ()  [unwired: 1 in, 1 out]
        n170 = flat-sequence {
          tunnel: w440 -> [w451]
          tunnel: w441 -> [w449]
          tunnel: [w450] -> w443
          tunnel: [w448] -> w442
          tunnel: [w464] -> w438
          tunnel: w443 -> [w467]
          tunnel: w442 -> [w466]
          tunnel: [w465] -> w439
          frame #0 {
            n171 = local read "Screen Index"() -> (w447:i32)
            n172 = case shown="-1, 2" w447 {
              selector: w447 -> [_ w459]
              tunnel: w451 -> [w453 w455]
              tunnel: [w453 w457] -> w450
              tunnel: w449 -> [w452 w458]
              tunnel: [w452 w458] -> w448
              frame -1, 2 {
              }
              frame 0, Default {
                n173 = invoke on="Sub Panel" class="SubPnl" method="Remove VI"(error in=w455) -> (error out=w454:errorcluster)  [unwired: 2 in, 2 out]
                n174 = Index Array(array=w458, index=w459) -> (element=w456:refnum<vi>)
                n175 = call "if VI is running stop VI.vi"("error in (no error)"=w454, "VI in"=w456) -> ("error out"=w457:errorcluster)  [unwired: 8 in, 1 out]
              }
            }
          }
          frame #1 {
            w465 = 2 ("index")
            n176 = Index Array(array=w466, index=w465) -> (element=w460:refnum<vi>)
            n177 = local write "Screen Index"(w465) -> ()
            n178 = property class="VI"(reference=w460, error in=w467) -> (reference out=w461:refnum<vi>, error out=w462:errorcluster, "Exec.State"=w463:T5)
            n179 = case shown="\"Run top level\"" w463 {
              tunnel: [w470 w475] -> w464
              tunnel: w462 -> [w469 w476]
              tunnel: w461 -> [w468 _]
              tunnel: w466 -> [_ w474]
              frame "Run top level" {
                n180 = invoke on="Sub Panel" class="SubPnl" method="Insert VI"(error in=w469, "VI Ref"=w468) -> (error out=w470:errorcluster)  [unwired: 2 in, 3 out]
              }
              frame "Idle", Default {
                n181 = Index Array(array=w474, index=6) -> (element=w473:refnum<vi>)
                n182 = call "if VI is idle run VI.vi"("error in (no error)"=w476, "VI in"=w473) -> ("error out"=w471:errorcluster, "VI out"=w477:refnum<vi>)  [unwired: 8 in]
                n183 = invoke on="Sub Panel" class="SubPnl" method="Insert VI"(error in=w471, "VI Ref"=w477) -> (error out=w475:errorcluster)  [unwired: 2 in, 3 out]
              }
            }
          }
        }
        n184 = call "Change menu button color as per screen index.vi"("error in (no error)"=w438, "Screen Index"=w439, "Array"=w444) -> ("error out"=w445:errorcluster)  [unwired: 8 in]
      }
      event "auto": Value Change {
        n185 = event-data() -> ()  [unwired: 1 in, 1 out]
        n186 = flat-sequence {
          tunnel: w483 -> [w491]
          tunnel: w482 -> [w489]
          tunnel: [w490] -> w486
          tunnel: [w488] -> w485
          tunnel: [w487] -> w484
          tunnel: [w505] -> w480
          tunnel: w486 -> [w503]
          tunnel: w485 -> [w507]
          tunnel: w484 -> [_]
          tunnel: [w506] -> w479
          frame #0 {
            n187 = local read "Screen Index"() -> (w487:i32)
            n188 = case shown="-1, 2" w487 {
              selector: w487 -> [_ w499]
              tunnel: w491 -> [w493 w495]
              tunnel: [w493 w497] -> w490
              tunnel: w489 -> [w492 w498]
              tunnel: [w492 w498] -> w488
              frame -1, 2 {
              }
              frame 0, Default {
                n189 = invoke on="Sub Panel" class="SubPnl" method="Remove VI"(error in=w495) -> (error out=w494:errorcluster)  [unwired: 2 in, 2 out]
                n190 = Index Array(array=w498, index=w499) -> (element=w496:refnum<vi>)
                n191 = call "if VI is running stop VI.vi"("error in (no error)"=w494, "VI in"=w496) -> ("error out"=w497:errorcluster)  [unwired: 8 in, 1 out]
              }
            }
          }
          frame #1 {
            n192 = Index Array(array=w507, index=4) -> (element=w501:refnum<vi>)
            n193 = property class="VI"(reference=w501, error in=w503) -> (error out=w502:errorcluster, "Exec.State"=w500:T5)  [unwired: 1 out]
            n194 = case shown="\"Idle\", Default" w500 {
              tunnel: w502 -> [w510 w515]
              tunnel: [w510 w512] -> w505
              tunnel: w507 -> [_ w516]
              tunnel: [7 w514] -> w506
              frame "Bad" {
                n195 = One Button Dialog(message="Manual Mode  is Running") -> ()  [unwired: 1 in, 1 out]
              }
              frame "Idle", Default {
                w514 = 2 ("index")
                n196 = local write "Screen Index"(w514) -> ()
                n197 = Index Array(array=w516, index=w514) -> (element=w517:refnum<vi>)
                n198 = call "if VI is idle run VI.vi"("error in (no error)"=w515, "VI in"=w517) -> ("error out"=w511:errorcluster, "VI out"=w513:refnum<vi>)  [unwired: 8 in]
                n199 = invoke on="Sub Panel" class="SubPnl" method="Insert VI"(error in=w511, "VI Ref"=w513) -> (error out=w512:errorcluster)  [unwired: 2 in, 3 out]
              }
            }
          }
        }
        n200 = call "Change menu button color as per screen index.vi"("error in (no error)"=w480, "Screen Index"=w479, "Array"=w481) -> ("error out"=w478:errorcluster)  [unwired: 8 in]
      }
      event "MANUAL": Value Change {
        n201 = event-data() -> ()  [unwired: 1 in, 1 out]
        n202 = invoke on="Sub Panel" class="SubPnl" method="Remove VI"(error in=w520) -> (error out=w524:errorcluster)  [unwired: 2 in, 2 out]
        n203 = flat-sequence {
          tunnel: w524 -> [w531]
          tunnel: w521 -> [w529]
          tunnel: [w530] -> w526
          tunnel: [w528] -> w525
          tunnel: [w548] -> w523
          tunnel: w526 -> [w540]
          tunnel: w525 -> [w546]
          tunnel: [w547] -> w522
          frame #0 {
            n204 = local read "Screen Index"() -> (w527:i32)
            n205 = case shown="-1, 2" w527 {
              selector: w527 -> [_ w538]
              tunnel: w531 -> [w533 w536]
              tunnel: [w533 w535] -> w530
              tunnel: w529 -> [w532 w537]
              tunnel: [w532 w537] -> w528
              frame -1, 2 {
              }
              frame 0, Default {
                n206 = Index Array(array=w537, index=w538) -> (element=w534:refnum<vi>)
                n207 = call "if VI is running stop VI.vi"("error in (no error)"=w536, "VI in"=w534) -> ("error out"=w535:errorcluster)  [unwired: 8 in, 1 out]
              }
            }
          }
          frame #1 {
            n208 = Index Array(array=w546, index=3) -> (element=w541:refnum<vi>)
            n209 = property class="VI"(reference=w541, error in=w540) -> (error out=w544:errorcluster, "Exec.State"=w543:T5)  [unwired: 1 out]
            n210 = case shown="\"Idle\", Default" w543 {
              tunnel: w544 -> [w549 w551]
              tunnel: [TRUE FALSE] -> w542
              tunnel: [w549 w551] -> w539
              frame "Idle", Default {
              }
              frame "Run top level", "Running" {
              }
            }
            n211 = case shown="True" w542 {
              tunnel: w546 -> [_ w562]
              tunnel: [w554 w561] -> w548
              tunnel: w539 -> [w554 w560]
              tunnel: [3 ("index") w556] -> w547
              frame False {
                n212 = One Button Dialog(message="Auto Cycle is Running Go to Auto Cycle and Press EXIT") -> ()  [unwired: 1 in, 1 out]
              }
              frame True {
                w556 = 4 ("index")
                n213 = Index Array(array=w562, index=w556) -> (element=w557:refnum<vi>)
                n214 = call "if VI is idle run VI.vi"("error in (no error)"=w560, "VI in"=w557) -> ("error out"=w559:errorcluster, "VI out"=w558:refnum<vi>)  [unwired: 8 in]
                n215 = local write "Screen Index"(w556) -> ()
                n216 = invoke on="Sub Panel" class="SubPnl" method="Insert VI"(error in=w559, "VI Ref"=w558) -> (error out=w561:errorcluster)  [unwired: 2 in, 3 out]
              }
            }
          }
        }
        n217 = call "Change menu button color as per screen index.vi"("error in (no error)"=w523, "Screen Index"=w522, "Array"=w519) -> ("error out"=w518:errorcluster)  [unwired: 8 in]
      }
      event "REPORT": Value Change {
        n218 = event-data() -> ()  [unwired: 1 in, 3 out]
        n219 = invoke on="Sub Panel" class="SubPnl" method="Remove VI"(error in=w563) -> (error out=w568:errorcluster)  [unwired: 2 in, 2 out]
        n220 = flat-sequence {
          tunnel: w568 -> [w577]
          tunnel: w571 -> [w574]
          tunnel: [w576] -> w570
          tunnel: [w573] -> w569
          tunnel: [w590] -> w566
          tunnel: w570 -> [w589]
          tunnel: w569 -> [w591]
          tunnel: [w585] -> w564
          frame #0 {
            n221 = local read "Screen Index"() -> (w575:i32)
            n222 = case shown="-1, 2" w575 {
              selector: w575 -> [_ w584]
              tunnel: w577 -> [w579 w582]
              tunnel: [w579 w581] -> w576
              tunnel: w574 -> [w578 w583]
              tunnel: [w578 w583] -> w573
              frame -1, 2 {
              }
              frame 0, Default {
                n223 = Index Array(array=w583, index=w584) -> (element=w580:refnum<vi>)
                n224 = call "if VI is running stop VI.vi"("error in (no error)"=w582, "VI in"=w580) -> ("error out"=w581:errorcluster)  [unwired: 8 in, 1 out]
              }
            }
          }
          frame #1 {
            w585 = 3 ("index")
            n225 = local write "Screen Index"(w585) -> ()
            n226 = Index Array(array=w591, index=w585) -> (element=w586:refnum<vi>)
            n227 = call "if VI is idle run VI.vi"("error in (no error)"=w589, "VI in"=w586) -> ("error out"=w588:errorcluster, "VI out"=w587:refnum<vi>)  [unwired: 8 in]
            n228 = invoke on="Sub Panel" class="SubPnl" method="Insert VI"(error in=w588, "VI Ref"=w587) -> (error out=w590:errorcluster)  [unwired: 2 in, 3 out]
          }
        }
        n229 = call "Change menu button color as per screen index.vi"("error in (no error)"=w566, "Screen Index"=w564, "Array"=w565) -> ("error out"=w567:errorcluster)  [unwired: 8 in]
      }
      event "andon": Value Change {
        n230 = event-data() -> ()  [unwired: 1 in, 3 out]
        n231 = invoke on="Sub Panel" class="SubPnl" method="Remove VI"(error in=w592) -> (error out=w597:errorcluster)  [unwired: 2 in, 2 out]
        n232 = flat-sequence {
          tunnel: w597 -> [w606]
          tunnel: w600 -> [w603]
          tunnel: [w605] -> w599
          tunnel: [w602] -> w598
          tunnel: [w619] -> w595
          tunnel: w599 -> [w618]
          tunnel: w598 -> [w620]
          tunnel: [w614] -> w594
          frame #0 {
            n233 = local read "Screen Index"() -> (w604:i32)
            n234 = case shown="-1, 2" w604 {
              selector: w604 -> [_ w613]
              tunnel: w606 -> [w608 w611]
              tunnel: [w608 w610] -> w605
              tunnel: w603 -> [w607 w612]
              tunnel: [w607 w612] -> w602
              frame -1, 2 {
              }
              frame 0, Default {
                n235 = Index Array(array=w612, index=w613) -> (element=w609:refnum<vi>)
                n236 = call "if VI is running stop VI.vi"("error in (no error)"=w611, "VI in"=w609) -> ("error out"=w610:errorcluster)  [unwired: 8 in, 1 out]
              }
            }
          }
          frame #1 {
            w614 = 6 ("index")
            n237 = local write "Screen Index"(w614) -> ()
            n238 = Index Array(array=w620, index=w614) -> (element=w615:refnum<vi>)
            n239 = call "if VI is idle run VI.vi"("error in (no error)"=w618, "VI in"=w615) -> ("error out"=w617:errorcluster, "VI out"=w616:refnum<vi>)  [unwired: 8 in]
            n240 = invoke on="Sub Panel" class="SubPnl" method="Insert VI"(error in=w617, "VI Ref"=w616) -> (error out=w619:errorcluster)  [unwired: 2 in, 3 out]
          }
        }
        n241 = call "Change menu button color as per screen index.vi"("error in (no error)"=w595, "Screen Index"=w594, "Array"=w593) -> ("error out"=w596:errorcluster)  [unwired: 8 in]
      }
      event "Hardware Setting": Value Change {
        n242 = event-data() -> ()  [unwired: 1 in, 3 out]
        n243 = invoke on="Sub Panel" class="SubPnl" method="Remove VI"(error in=w621) -> (error out=w626:errorcluster)  [unwired: 2 in, 2 out]
        n244 = flat-sequence {
          tunnel: w626 -> [w635]
          tunnel: w629 -> [w632]
          tunnel: [w634] -> w628
          tunnel: [w631] -> w627
          tunnel: [w648] -> w624
          tunnel: w628 -> [w647]
          tunnel: w627 -> [w649]
          tunnel: [w643] -> w623
          frame #0 {
            n245 = local read "Screen Index"() -> (w633:i32)
            n246 = case shown="-1, 2" w633 {
              selector: w633 -> [_ w642]
              tunnel: w635 -> [w637 w640]
              tunnel: [w637 w639] -> w634
              tunnel: w632 -> [w636 w641]
              tunnel: [w636 w641] -> w631
              frame -1, 2 {
              }
              frame 0, Default {
                n247 = Index Array(array=w641, index=w642) -> (element=w638:refnum<vi>)
                n248 = call "if VI is running stop VI.vi"("error in (no error)"=w640, "VI in"=w638) -> ("error out"=w639:errorcluster)  [unwired: 8 in, 1 out]
              }
            }
          }
          frame #1 {
            w643 = 4 ("index")
            n249 = local write "Screen Index"(w643) -> ()
            n250 = Index Array(array=w649, index=w643) -> (element=w644:refnum<vi>)
            n251 = call "if VI is idle run VI.vi"("error in (no error)"=w647, "VI in"=w644) -> ("error out"=w646:errorcluster, "VI out"=w645:refnum<vi>)  [unwired: 8 in]
            n252 = invoke on="Sub Panel" class="SubPnl" method="Insert VI"(error in=w646, "VI Ref"=w645) -> (error out=w648:errorcluster)  [unwired: 2 in, 3 out]
          }
        }
        n253 = call "Change menu button color as per screen index.vi"("error in (no error)"=w624, "Screen Index"=w623, "Array"=w622) -> ("error out"=w625:errorcluster)  [unwired: 8 in]
      }
      event "Shift Setting": Value Change {
        n254 = event-data() -> ()  [unwired: 1 in, 3 out]
        n255 = invoke on="Sub Panel" class="SubPnl" method="Remove VI"(error in=w650) -> (error out=w655:errorcluster)  [unwired: 2 in, 2 out]
        n256 = flat-sequence {
          tunnel: w655 -> [w664]
          tunnel: w658 -> [w661]
          tunnel: [w663] -> w657
          tunnel: [w660] -> w656
          tunnel: [w677] -> w651
          tunnel: w657 -> [w676]
          tunnel: w656 -> [w678]
          tunnel: [w672] -> w653
          frame #0 {
            n257 = local read "Screen Index"() -> (w662:i32)
            n258 = case shown="-1, 2" w662 {
              selector: w662 -> [_ w671]
              tunnel: w664 -> [w666 w669]
              tunnel: [w666 w668] -> w663
              tunnel: w661 -> [w665 w670]
              tunnel: [w665 w670] -> w660
              frame -1, 2 {
              }
              frame 0, Default {
                n259 = Index Array(array=w670, index=w671) -> (element=w667:refnum<vi>)
                n260 = call "if VI is running stop VI.vi"("error in (no error)"=w669, "VI in"=w667) -> ("error out"=w668:errorcluster)  [unwired: 8 in, 1 out]
              }
            }
          }
          frame #1 {
            w672 = 5 ("index")
            n261 = local write "Screen Index"(w672) -> ()
            n262 = Index Array(array=w678, index=w672) -> (element=w673:refnum<vi>)
            n263 = call "if VI is idle run VI.vi"("error in (no error)"=w676, "VI in"=w673) -> ("error out"=w675:errorcluster, "VI out"=w674:refnum<vi>)  [unwired: 8 in]
            n264 = invoke on="Sub Panel" class="SubPnl" method="Insert VI"(error in=w675, "VI Ref"=w674) -> (error out=w677:errorcluster)  [unwired: 2 in, 3 out]
          }
        }
        n265 = call "Change menu button color as per screen index.vi"("error in (no error)"=w651, "Screen Index"=w653, "Array"=w652) -> ("error out"=w654:errorcluster)  [unwired: 8 in]
      }
      event "Test Print": Value Change {
        n266 = event-data() -> ()  [unwired: 1 in, 3 out]
        n267 = invoke on="Sub Panel" class="SubPnl" method="Remove VI"(error in=w679) -> (error out=w684:errorcluster)  [unwired: 2 in, 2 out]
        n268 = flat-sequence {
          tunnel: w684 -> [w693]
          tunnel: w687 -> [w690]
          tunnel: [w692] -> w686
          tunnel: [w689] -> w685
          tunnel: [w706] -> w682
          tunnel: w686 -> [w705]
          tunnel: w685 -> [w707]
          tunnel: [w701] -> w681
          frame #0 {
            n269 = local read "Screen Index"() -> (w691:i32)
            n270 = case shown="-1, 2" w691 {
              selector: w691 -> [_ w700]
              tunnel: w693 -> [w695 w698]
              tunnel: [w695 w697] -> w692
              tunnel: w690 -> [w694 w699]
              tunnel: [w694 w699] -> w689
              frame -1, 2 {
              }
              frame 0, Default {
                n271 = Index Array(array=w699, index=w700) -> (element=w696:refnum<vi>)
                n272 = call "if VI is running stop VI.vi"("error in (no error)"=w698, "VI in"=w696) -> ("error out"=w697:errorcluster)  [unwired: 8 in, 1 out]
              }
            }
          }
          frame #1 {
            w701 = 9 ("index")
            n273 = local write "Screen Index"(w701) -> ()
            n274 = Index Array(array=w707, index=w701) -> (element=w702:refnum<vi>)
            n275 = call "if VI is idle run VI.vi"("error in (no error)"=w705, "VI in"=w702) -> ("error out"=w704:errorcluster, "VI out"=w703:refnum<vi>)  [unwired: 8 in]
            n276 = invoke on="Sub Panel" class="SubPnl" method="Insert VI"(error in=w704, "VI Ref"=w703) -> (error out=w706:errorcluster)  [unwired: 2 in, 3 out]
          }
        }
        n277 = call "Change menu button color as per screen index.vi"("error in (no error)"=w682, "Screen Index"=w681, "Array"=w680) -> ("error out"=w683:errorcluster)  [unwired: 8 in]
      }
      event "Home": Value Change {
        n278 = event-data() -> ()  [unwired: 1 in, 3 out]
        n279 = invoke on="Sub Panel" class="SubPnl" method="Remove VI"(error in=w708) -> (error out=w711:errorcluster)  [unwired: 2 in, 2 out]
        n280 = call "Change menu button color as per screen index.vi"("error in (no error)"=w711, "Screen Index"=-1, "Array"=w709) -> ("error out"=w710:errorcluster)  [unwired: 8 in]
      }
      event "EXIT": Value Change {
        n281 = event-data() -> ()  [unwired: 1 in, 1 out]
        n282 = Index Array(array=w716, index=2) -> (element=w722:refnum<vi>)
        n283 = Build Array(w722) -> (w721:refnum<vi>[])
        n284 = for {
          tunnel: w716 -> [w745]
          tunnel: [w744] -> w724 mode=indexing
          shift-right: [w743] -> w718
          shift-left: w723 -> [w742]
          tunnel: w721 -> [w741] mode=indexing
          n285 = property class="VI"(reference=w741, error in=w742) -> (error out=w747:errorcluster, "Exec.State"=w746:T5)  [unwired: 1 out]
          n286 = case shown="\"Run top level\", \"Running\"" w746 {
            tunnel: w747 -> [w748 w750]
            tunnel: w745 -> [_ _]
            tunnel: [TRUE FALSE] -> w744
            tunnel: [w748 w750] -> w743
            frame "Idle", Default {
            }
            frame "Run top level", "Running" {
            }
          }
        }
        n287 = And Array Elements(Boolean array=w724) -> (logical AND=w720:bool)
        n288 = case shown="False" w720 {
          tunnel: [FALSE TRUE] -> w715
          tunnel: w718 -> [w729 w733]
          tunnel: [w729 w732] -> w717
          tunnel: w716 -> [_ w731]
          frame False {
            n289 = One Button Dialog(message="Auto Cycle  is Running") -> ()  [unwired: 1 in, 1 out]
          }
          frame True {
            n290 = invoke on="Sub Panel" class="SubPnl" method="Remove VI"(error in=w733) -> (error out=w734:errorcluster)  [unwired: 2 in, 2 out]
            n291 = for {
              shift-right: [w740] -> w732
              shift-left: w734 -> [w739]
              tunnel: w731 -> [w735] mode=indexing
              n292 = call "if VI is running stop VI.vi"("error in (no error)"=w739, "VI in"=w735) -> ("error out"=w738:errorcluster, "VI out"=w737:refnum<vi>)  [unwired: 8 in]
              n293 = call <vilib>:"Clear Errors.vi"("error in (no error)"=w738) -> ("error out"=w736:errorcluster)  [unwired: 5 in, 1 out]
              n294 = Close Reference(reference=w737, error in (no error)=w736) -> (error out=w740:errorcluster)
            }
          }
        }
        n295 = call "Change menu button color as per screen index.vi"("error in (no error)"=w717, "Screen Index"=-1, "Array"=w719) -> ("error out"=w714:errorcluster)  [unwired: 8 in]
      }
      event "Remove": Value Change {
        n296 = event-data() -> ()  [unwired: 1 in, 1 out]
        n297 = invoke on="Sub Panel" class="SubPnl" method="Remove VI"(error in=w752) -> (error out=w754:errorcluster)  [unwired: 2 in, 2 out]
        n298 = call "Change menu button color as per screen index.vi"("error in (no error)"=w754, "Screen Index"=-1, "Array"=w753) -> ("error out"=w755:errorcluster)  [unwired: 8 in]
      }
      event Timeout {
        n299 = event-data() -> ()  [unwired: 1 in, 1 out]
        n300 = global read "Global 1.vi" "MODEL SELECTION"() -> (w768:bool)
        n301 = global read "Global 1.vi" "BARCODE RECIPE"() -> (w767:string)
        n302 = Format Date/Time String(time format string (%c)="%d/ %m/ %Y\n%H:%M:%S") -> (date/time string=→"datetime":string)  [unwired: 2 in]
        n303 = global read "Login Details.vi" "User Name"() -> (→"user name":string)
        n304 = Empty String/Path?(string/path=w767) -> (empty?=w766:bool)
        n305 = Or(x="Check 2", y=w768) -> (x .or. y?=w772:bool)
        n306 = case shown="True" w772 {
          tunnel: w770 -> [w800 w805]
          tunnel: [w800 w804] -> w759
          tunnel: w766 -> [_ w802]
          frame False {
          }
          frame True {
            n307 = flat-sequence {
              tunnel: w805 -> [w809]
              tunnel: [w807] -> w803
              tunnel: w802 -> [w806]
              tunnel: [w806] -> w801
              tunnel: [w812] -> w804
              tunnel: w803 -> [w813]
              tunnel: w801 -> [w811]
              frame #0 {
                n308 = invoke on="Sub Panel" class="SubPnl" method="Remove VI"(error in=w809) -> (error out=w807:errorcluster)  [unwired: 2 in, 2 out]
                n309 = global write "Global 1.vi" "MODEL SELECTION"(FALSE ("remove_VI")) -> ()
                n310 = local write "Check 2"(FALSE ("Check")) -> ()
              }
              frame #1 {
                n311 = case shown="False" w811 {
                  tunnel: w813 -> [w815 w817]
                  tunnel: [w814 w817] -> w812
                  frame False {
                    n312 = property on="auto" class="Bool (strict)"(error in=w815, "Val(Sgnl)"=TRUE ("Value (Signaling)")) -> (error out=w814:errorcluster)  [unwired: 1 in, 1 out]
                  }
                  frame True {
                  }
                }
              }
            }
          }
        }
        n313 = control-ref of="Hardware Setting"() -> (w762:refnum<vi>)
        n314 = control-ref of="Shift Setting"() -> (w761:refnum<vi>)
        n315 = control-ref of="REPORT"() -> (w763:refnum<vi>)
        n316 = control-ref of="USER MANGMENT"() -> (w765:refnum<vi>)
        n317 = control-ref of="AUTO MODE"() -> (w764:refnum<vi>)
        n318 = Build Array(w765, w764, w763, w762, w761) -> (w760:refnum<vi>[])
        n319 = global read "Login Details.vi" "Authority"() -> (w793:T2)
        n320 = Unbundle By Name(w793) -> ("SCREEN 2"=w791:bool, "SCREEN 3"=w790:bool, "SCREEN 4"=w789:bool, "SCREEN 5"=w788:bool, "SCREEN 6"=w787:bool, "SCREEN 7"=w786:bool, "SCREEN 8"=w785:bool, "SCREEN 9"=w784:bool, "SCREEN 10"=w783:bool, "SCREEN 11"=w782:bool, "SCREEN 12"=w781:bool, "SCREEN 13"=w780:bool, "SCREEN 14"=w779:bool, "SCREEN 15"=w778:bool, "SCREEN 16"=w777:bool, "SCREEN 17"=w776:bool, "SCREEN 18"=w775:bool, "SCREEN 19"=w774:bool, "SCREEN 20"=w773:bool)  [unwired: 1 out]
        n321 = Build Array(w791, w790, w789, w788, w787, w786, w785, w784, w783, w782, w781, w780, w779, w778, w777, w776, w775, w774, w773) -> (w792:bool[])
        n322 = for {
          tunnel: w792 -> [w820] mode=indexing
          tunnel: w760 -> [w821] mode=indexing
          tunnel: w759 -> [w819]
          tunnel: [w818] -> w758
          n323 = case shown="True" w820 {
            tunnel: w821 -> [w824 w828]
            tunnel: w819 -> [w823 w827]
            tunnel: [w822 w826] -> w818
            frame True {
              n324 = property class="Bool"(reference=w824, error in=w823, "DisabledEnum"=T3."Enabled" ("Disabled")) -> (error out=w822:errorcluster)  [unwired: 1 out]
            }
            frame False {
              n325 = property class="Bool"(reference=w828, error in=w827, "DisabledEnum"=T3."Disabled and Grayed Out" ("Disabled")) -> (error out=w826:errorcluster)  [unwired: 1 out]
            }
          }
        }
        n326 = global read "Global 1.vi" "REMOVE VI"() -> (w769:bool)
        n327 = Or(x="Check", y=w769) -> (x .or. y?=w797:bool)
        n328 = case shown="True" w797 {
          selector: w797 -> [_ w832]
          frame False {
          }
          frame True {
            n329 = global write "Global 1.vi" "REMOVE VI"(FALSE ("remove_VI")) -> ()
            n330 = property on="Remove" class="Bool (strict)"("Val(Sgnl)"=w832) -> ()  [unwired: 2 in, 2 out]
            n331 = local write "Check"(FALSE ("Check")) -> ()
          }
        }
      }
    }
  }
  n332 = call <vilib>:"Clear Errors.vi"("error in (no error)"=w22) -> ("error out"=w12:errorcluster)  [unwired: 5 in, 1 out]
  n333 = disable-structure shown="Disabled" {
    disable-tunnel: w1 -> [w833 _]
    frame Disabled {
      n334 = Quit LabVIEW(quit? (T)=w833) -> ()
    }
    frame Enabled {
    }
  }
  n335 = call "PADMINI_STOP_ALL.vi"("Enum"=enum16{"Read", "Write"}."Write", "error in (no error)"=w12, "Boolean"=TRUE) -> ("error out"=w9:errorcluster)  [unwired: 7 in, 1 out]
  n336 = call <vilib>:"Clear Errors.vi"("error in (no error)"=w9) -> ("error out"=w35:errorcluster)  [unwired: 5 in, 1 out]
  n337 = property class="App"(error in=w35) -> (error out=w36:errorcluster, "App.Kind"=w37:T6)  [unwired: 1 in, 1 out]
  n338 = case shown="\"Run Time System\"" w37 {
    tunnel: w36 -> [w834 w836]
    tunnel: [w834 w835] -> w34
    frame Default {
    }
    frame "Run Time System" {
      n339 = invoke class="VI" method="FP.Close"(error in=w836) -> (error out=w835:errorcluster)  [unwired: 2 in, 2 out]
    }
  }
  "error out 2" <- w34
